vi "Associated Research 78XX Series Editing Steps Within a File.vi"(8 "error in (no error)":errorcluster, 11 "VISA resource name":refnum<visa-resource-name>) -> (0 "error out":errorcluster)   [LabVIEW 2012]
doc: "This VI is an example of how to edit steps. This will take previously created file \"RandomT\" and edit the IR parameters.\nNOTE: \"Creating and Saving a File\" is required to run before this VI."
uses:
  <instrlib>/Associated Research 78XX Series/Public/Configure/Steps/Low Level/IR Test Parameters.ctl
  <instrlib>/Associated Research 78XX Series/Public/Configure/Steps/Low Level/Scanner Settings.ctl
  <instrlib>/Associated Research 78XX Series/Associated Research 78XX Series.lvlib
panel:
  in  "Internal Scanner Exists?":bool
  in  "Scanner Settings":T1={"Scan1"=1, "Scan2"=1, "Scan3"=1, "Scan4"=1, "Scan5"=1, "Scan6"=1, "Scan7"=1, "Scan8"=1, "Scan9"=1, "Scan10"=1, "Scan11"=1, "Scan12"=1, "Scan13"=1, "Scan14"=1, "Scan15"=1, "Scan16"=1} {"Scan16" scale=0.0..2.0; "Scan15" scale=0.0..2.0; "Scan14" scale=0.0..2.0; "Scan13" scale=0.0..2.0; "Scan12" scale=0.0..2.0; "Scan11" scale=0.0..2.0; "Scan10" scale=0.0..2.0; "Scan9" scale=0.0..2.0; "Scan8" scale=0.0..2.0; "Scan7" scale=0.0..2.0; "Scan6" scale=0.0..2.0; "Scan5" scale=0.0..2.0; "Scan4" scale=0.0..2.0; "Scan3" min=0 max=2 scale=0.0..2.0; "Scan2" min=0 max=2 scale=0.0..2.0; "Scan1" min=0 max=2 scale=0.0..2.0}
  in  "IR Test Parameters in":T2={"Voltage (1000)"=1000, "High Limit(0.0, 0.5 - 50000 Megohms) (5)"=0.0, "Low Limit(0.1 - 50000 Megohms) (0)"=0.1, "Ramp Up Time (0.1 - 999.9 seconds) (0.1)"=0.1, "Delay Time (0.0, 1.0 - 999.9 seconds) (0.5)"=0.5, "Ramp Down Time (0.0 - 999.9 seconds) (0) "=0.0, "Charge LO (0)"=0.0, "Auto Charge LO (F: Off)"=FALSE, "Dwell Time (0.0, 1.0 - 999.9 seconds) (0.5)"=0.5} {"Dwell Time (0.0, 1.0 - 999.9 seconds) (0.5)" format="%.1f"; "Ramp Down Time (0.0 - 999.9 seconds) (0)" format="%.1f"; "Charge LO (0)" format="%.2f"; "Delay Time (0.0, 1.0 - 999.9 seconds) (0.5)" format="%.1f"; "Ramp Up Time (0.1 - 999.9 seconds) (0.1)" format="%.1f"; "Low Limit(0.1 - 50000 Megohms) (0)" format="%.1f"; "High Limit(0.0, 0.5 - 50000 Megohms) (5)" format="%.1f"}
  out "Step Parameters":string
  out "Number of Steps (0)":i32
  out "error Occured?":bool
  # "On\nOff"
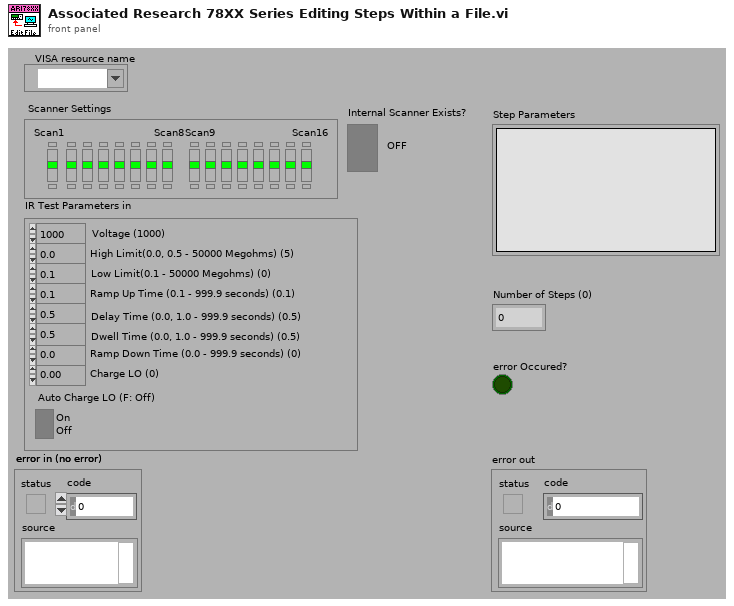
[diagram p1: front panel]
types:
  T1 = typedef "Associated Research 78XX Series.lvlib/Scanner Settings.ctl" = cluster{"Scan1":i32, "Scan2":i32, "Scan3":i32, "Scan4":i32, "Scan5":i32, "Scan6":i32, "Scan7":i32, "Scan8":i32, "Scan9":i32, "Scan10":i32, "Scan11":i32, "Scan12":i32, "Scan13":i32, "Scan14":i32, "Scan15":i32, "Scan16":i32}
  T2 = typedef "Associated Research 78XX Series.lvlib/IR Test Parameters.ctl" = cluster{"Voltage (1000)":i32, "High Limit(0.0, 0.5 - 50000 Megohms) (5)":dbl, "Low Limit(0.1 - 50000 Megohms) (0)":dbl, "Ramp Up Time (0.1 - 999.9 seconds) (0.1)":dbl, "Delay Time (0.0, 1.0 - 999.9 seconds) (0.5)":dbl, "Ramp Down Time (0.0 - 999.9 seconds) (0) ":dbl, "Charge LO (0)":dbl, "Auto Charge LO (F: Off)":bool, "Dwell Time (0.0, 1.0 - 999.9 seconds) (0.5)":dbl}
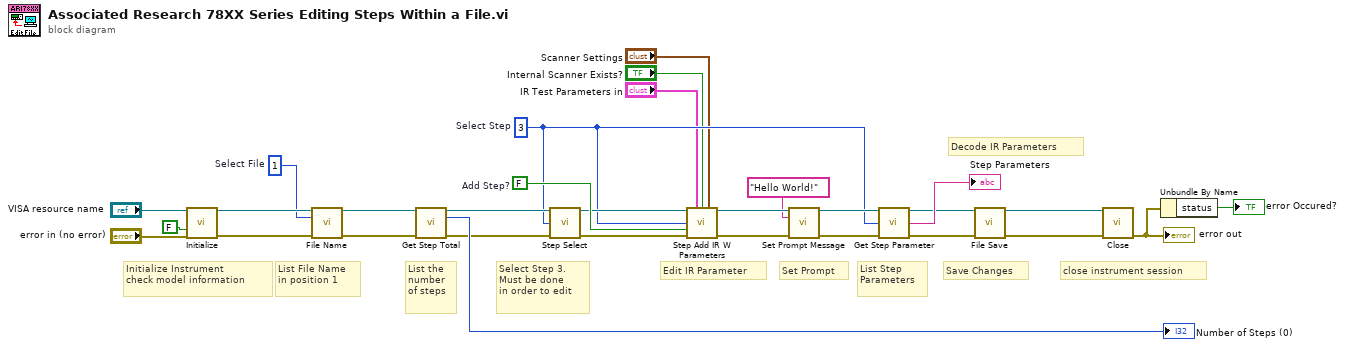
[diagram p0: block diagram]
diagram:
  w4 = 3  # Select Step
  w16 = FALSE  # Add Step?
  w23 = 1  # Select File
  # "Save Changes"
  # "List Step\nParameters"
  # "Set Prompt"
  # "Edit IR Parameter"
  # "Select Step 3.\nMust be done\nin order to edit"
  # "List the\nnumber\nof steps"
  # "close instrument session"
  # "Decode IR Parameters"
  # "List File Name\nin position 1"
  # "Initialize Instrument \ncheck model information"
  n1 = call <instrlib>:"Initialize.vi"("VISA resource name"="VISA resource name", "Reset (True)"=FALSE, "error in (no error)"="error in (no error)") -> ("VISA resource name out"=w25:refnum<visa-resource-name>, "error out"=w24:errorcluster)  [unwired: 10 in, 1 out]
  n2 = call <instrlib>:"File Name.vi"("VISA resource name"=w25, "File Number"=w23, "error in (no error)"=w24) -> ("VISA resource name out"=w22:refnum<visa-resource-name>, "error out"=w21:errorcluster)  [unwired: 10 in, 1 out]
  n3 = call <instrlib>:"Get Step Total.vi"("VISA resource name"=w22, "error in (no error)"=w21) -> ("VISA resource name out"=w15:refnum<visa-resource-name>, "# of Steps"=→"Number of Steps (0)":i32, "error out"=w14:errorcluster)  [unwired: 11 in]
  n4 = call <instrlib>:"Step Select.vi"("VISA resource name"=w15, "Step Number (1)"=w4, "error in (no error)"=w14) -> ("VISA resource name out"=w13:refnum<visa-resource-name>, "error out"=w12:errorcluster)  [unwired: 11 in]
  n5 = call <instrlib>:"Step Add IR W Parameters.vi"("VISA resource name"=w13, "IR Test Parameters in"="IR Test Parameters in", "Internal Scanner Exists?"="Internal Scanner Exists?", "Scanner Settings"="Scanner Settings", "Step Selection (1-200)"=w4, "Add Step"=w16, "error in (no error)"=w12) -> ("VISA resource name out"=w11:refnum<visa-resource-name>, "error out"=w10:errorcluster)  [unwired: 7 in]
  n6 = call <instrlib>:"Set Prompt Message.vi"("VISA resource name"=w11, "Prompt (empty)"="Hello World!", "error in (no error)"=w10) -> ("VISA resource name out"=w9:refnum<visa-resource-name>, "error out"=w7:errorcluster)  [unwired: 11 in]
  n7 = call <instrlib>:"Get Step Parameter.vi"("VISA resource name"=w9, "Step Number (0 = Active Step)"=w4, "error in (no error)"=w7) -> ("VISA resource name out"=w8:refnum<visa-resource-name>, "Step Parameter"=→"Step Parameters":string, "error out"=w6:errorcluster)  [unwired: 10 in]
  n8 = call <instrlib>:"File Save.vi"("VISA resource name"=w8, "error in (no error)"=w6) -> ("VISA resource name out"=w19:refnum<visa-resource-name>, "error out"=w20:errorcluster)  [unwired: 12 in]
  n9 = call <instrlib>:"Close.vi"("VISA resource name"=w19, "error in (no error)"=w20) -> ("error out"=w26:errorcluster)  [unwired: 13 in]
  "error out" <- w26
  n10 = Unbundle By Name(w26) -> ("status"=→"error Occured?":bool)
